vi "Read Name.vi"(8 "error in (no error)":errorcluster, 11 "Process In":refnum<class "Process.lvclass">) -> (0 "error out":errorcluster, 1 "Name":string, 2 "Qualified Name":string, 3 "Process Out":refnum<class "Process.lvclass">)   [LabVIEW 2020, in "Process.lvclass"]
doc: "Returns the name of the object. The Qualified Name is prepended with the name of the owner recursively in the format \"Owner Name::Name\"."
uses:
  Process.lvclass
  Process.lvclass/Process.ctl
  <vilib>/Utility/error.llb/Error Cluster From Error Code.vi
  Application/Application.lvclass
  Base/Base.lvclass
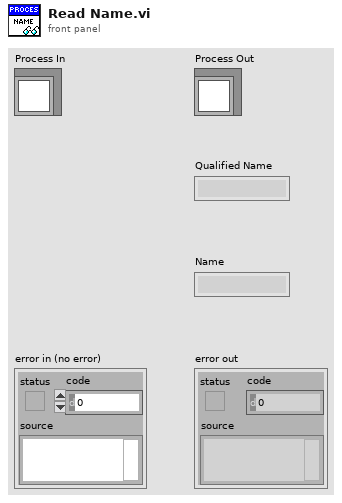
[diagram p1: front panel]
types:
  T1 = typedef "Process.lvclass/Lifecycle State.ctl" = enum16{"Uninitialized", "Initialized", "Started", "Running", "Stopped", "Finished"}
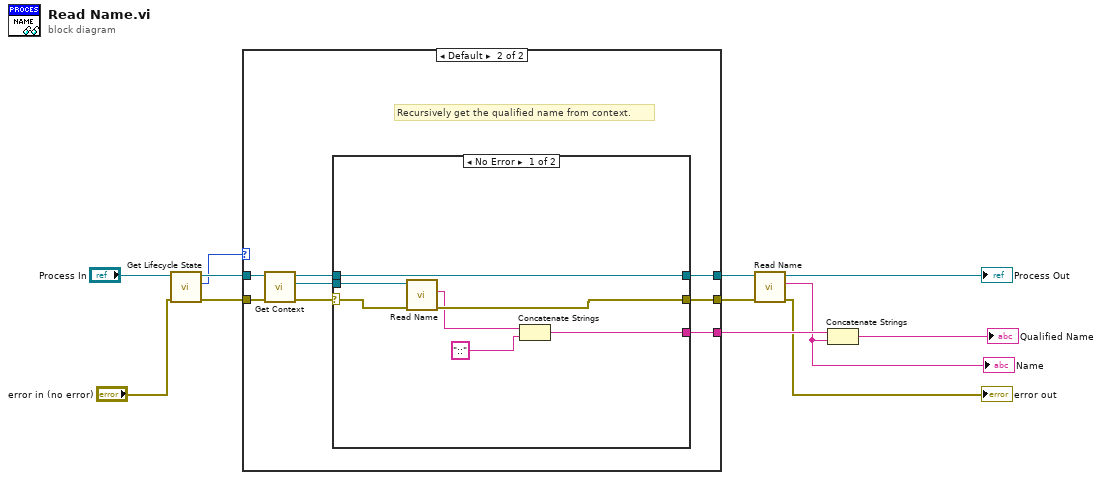
[diagram p0: block diagram]
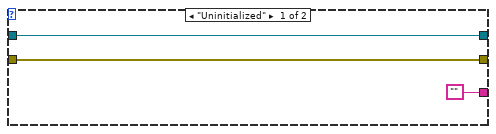
[diagram p2: hidden frame]
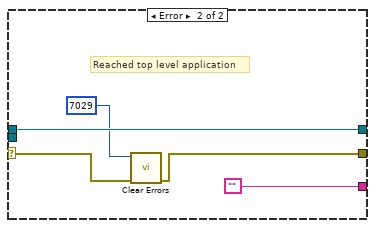
[diagram p3: hidden frame]
diagram:
  n1 = call "Get Lifecycle State.vi"("error in (no error)"="error in (no error)", "Process In"="Process In") -> ("error out"=w2:errorcluster, "Lifecycle State"=w1:T1, "Process Out"=w4:refnum<class "Process.lvclass">)  [unwired: 6 in, 1 out]
  n2 = case shown="Default" w1 {
    tunnel: [w15 w23] -> w11
    tunnel: ["" w19] -> w9
    tunnel: [w14 w18] -> w6
    tunnel: w4 -> [w15 w17]
    tunnel: w2 -> [w14 w16]
    frame "Uninitialized" {
    }
    frame Default {
      # "Recursively get the qualified name from context."
      n3 = call "Get Context.vi"("error in (no error)"=w16, "Process In"=w17) -> ("error out"=w22:errorcluster, "Context"=w21:refnum<class "Application.lvclass">, "Process Out"=w20:refnum<class "Process.lvclass">)  [unwired: 7 in]
      n4 = case shown="No Error" w22 {
        selector: w22 -> [w28 w32]
        tunnel: w21 -> [w30 _]
        tunnel: w20 -> [w29 w35]
        tunnel: [w27 w31] -> w18
        tunnel: [w29 w35] -> w23
        tunnel: [w25 ""] -> w19
        frame No Error {
          n5 = call-dynamic "Read Name.vi"("error in (no error)"=w28, "Process In"=w30) -> ("error out"=w27:errorcluster, "Qualified Name"=w24:string)  [unwired: 6 in, 2 out]
          n6 = Concatenate Strings(w24, "::" ("delimiter")) -> (w25:string)
        }
        frame Error {
          # "Reached top level application"
          n7 = call <vilib>:"Clear Errors.vi"("error in (no error)"=w32, "specific error code to clear (0: all)"=7029) -> ("error out"=w31:errorcluster)  [unwired: 4 in, 1 out]
        }
      }
    }
  }
  n8 = call-parent "Read Name.vi"("error in (no error)"=w6, "Base In"=w11) -> ("error out"=→"error out":errorcluster, "Qualified Name"=w8:string, "Base Out"=→"Process Out":refnum<class "Process.lvclass">)  [unwired: 6 in, 1 out]
  "Name" <- w8
  n9 = Concatenate Strings(w9, w8) -> (→"Qualified Name":string)
